vi "PH_Beckhoff_Watchdog.ProcCases.vi"(0 "i ref in":refnum<vi>, 1 "selector":string, 2 "Data":T1, 3 "call cluster":T2={"Object"="", "Selector"="", "CallType"=enum."synchronous", "Async Object"="", "Async Selector"="", "Data Descriptor"="", "Data"=[], "Error #"=0, "Expire"=0}, 5 "error in (no error)":errorcluster) -> (14 "i ref out":refnum<vi>, 17 "answer cluster":T2={"Object"="", "Selector"="", "CallType"=enum."synchronous", "Async Object"="", "Async Selector"="", "Data Descriptor"="", "Data"=[], "Error #"=0, "Expire"=0}, 19 "error out":errorcluster)   [LabVIEW 2014, in "PH_Beckhoff_Watchdog.lvlib"]
doc: "This method is called by a process from within the default case in the event loop. The methods of a class that are linked to events will be called from THIS method. Add your code here."
uses:
  PH_Beckhoff_Watchdog.lvlib
  CSCore/CSSystem/CoreDefs/CoreDefs.call_type.ctl
  CSCore/BaseProcess/BaseProcess.descriptor string definition.ctl
  CSCore/CSSystem/CoreDefs/CoreDefs.rawDataType.ctl
  CSCore/CSSystem/CoreLib/CoreLib.string 2 byte array.vi
  CSCore/BaseProcess/BaseProcess.lvlib
  CSCore/CSSystem/CoreLib/CoreLib.lvlib
  CSCore/CAEObj/CAEObj.lvlib
  PH_Common/PH_Common.lvlib
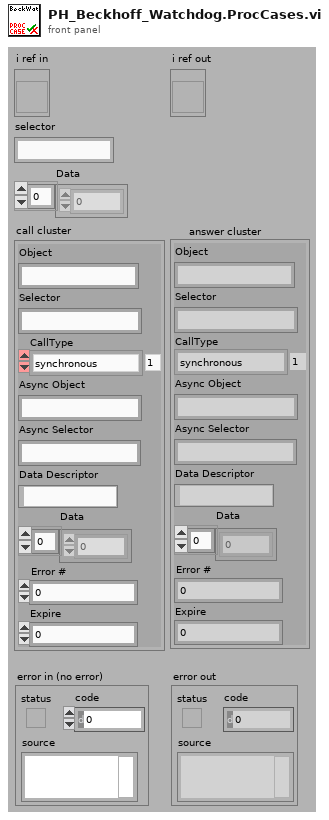
[diagram p1: front panel]
types:
  T1 = typedef "CoreDefs.rawDataType.ctl" = i8[]
  T2 = typedef "CoreDefs.call_type.ctl" = cluster{"Object":string, "Selector":string, "CallType":enum16{"simple", "synchronous", "asynchronous"}, "Async Object":string, "Async Selector":string, "Data Descriptor":T3, "Data":T1, "Error #":i32, "Expire":u32}
  T3 = typedef "BaseProcess.lvlib/BaseProcess.descriptor string definition.ctl" = string
  T4 = typedef "PH_StatusHandler.lvlib/PH_StatusHandler.Status.ctl" = i16
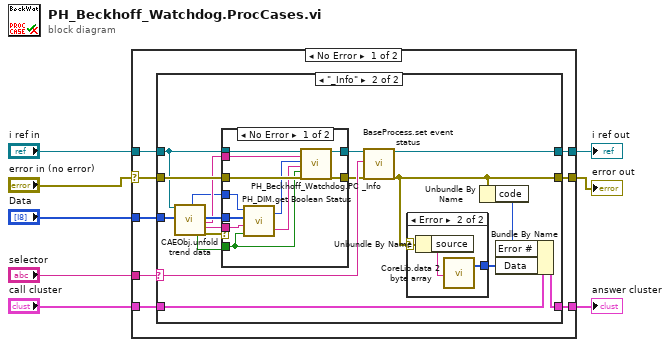
[diagram p0: block diagram]
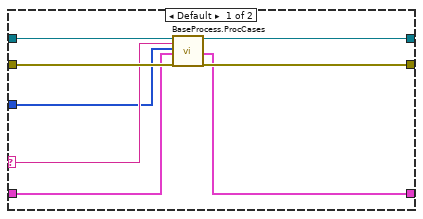
[diagram p2: hidden frame]
diagram:
  n1 = case shown="No Error" "error in (no error)" {
    selector: "error in (no error)" -> [w9 w60]
    tunnel: "selector" -> [w16 _]
    tunnel: [w15 w59] -> w7
    tunnel: "call cluster" -> [w14 w59]
    tunnel: "i ref in" -> [w13 w61]
    tunnel: [w12 w61] -> w4
    tunnel: [w11 w60] -> w3
    tunnel: "Data" -> [w10 _]
    frame No Error {
      n2 = case shown="\"_Info\"" w16 {
        selector: w16 -> [w19 w41]
        tunnel: w13 -> [w18 w31]
        tunnel: [w24 w40] -> w12
        tunnel: w14 -> [w20 w38]
        tunnel: [w21 w37] -> w15
        tunnel: w9 -> [w23 w36]
        tunnel: [w22 w39] -> w11
        tunnel: w10 -> [w17 w32]
        frame Default {
          n3 = call "BaseProcess.ProcCases.vi"("i ref in"=w18, "selector"=w19, "Data"=w17, "call cluster"=w20, "error in (no error)"=w23) -> ("i ref out"=w24:refnum<vi>, "answer cluster"=w21:T2, "error out"=w22:errorcluster)  [unwired: 12 in]
        }
        frame "_Info" {
          n4 = call "CAEObj.unfold trend data.vi"("i ref in"=w31, "raw trend data"=w32) -> ("quality"=w26:i32, "no link"=w28:bool, "data"=w29:i8[], "serviceName"=w27:string, "typeDescriptor"=w25:string, "error out"=w30:errorcluster)  [unwired: 9 in, 3 out]
          n5 = case shown="No Error" w30 {
            tunnel: w36 -> [w53 w54]
            tunnel: [w52 w55] -> w35
            tunnel: [w51 w54] -> w34
            tunnel: w31 -> [w50 w55]
            tunnel: w25 -> [w49 _]
            tunnel: w29 -> [w48 _]
            tunnel: w28 -> [w43 _]
            tunnel: w27 -> [w47 _]
            tunnel: w26 -> [w46 _]
            frame No Error {
              n6 = call "PH_DIM.get Boolean Status.vi"("no link"=w43, "typeDescriptor"=w49, "data"=w48, "quality"=w46) -> ("further information"=w45:string, "Status"=w44:T4)
              n7 = call "PH_Beckhoff_Watchdog.PC _Info.vi"("i ref in"=w50, "serviceName"=w47, "Status"=w44, "Further Information"=w45, "no link"=w43, "error in"=w53) -> ("i ref out"=w52:refnum<vi>, "error out"=w51:errorcluster)  [unwired: 12 in]
            }
            frame Error {
            }
          }
          n8 = call "BaseProcess.set event status.vi"("i ref in"=w35, "EventStatus"=w41, "error in (no error)"=w34) -> ("i ref out"=w40:refnum<vi>, "error out"=w39:errorcluster)  [unwired: 14 in, 1 out]
          n9 = case shown="Error" w39 {
            selector: w39 -> [_ w58]
            tunnel: [_ w56] -> w42
            frame No Error {
            }
            frame Error {
              n10 = Unbundle By Name(w58) -> ("source"=w57:string)
              n11 = call-poly "CoreLib.data 2 byte array.vi"("string"=w57) -> ("byteArray out"=w56:T1)  [unwired: 18 in]
            }
          }
          n12 = Unbundle By Name(w39) -> ("code"=w33:i32)
          n13 = Bundle By Name(cluster=w38, "Error #"=w33, "Data"=w42) -> (w37:T2)
        }
      }
    }
    frame Error {
    }
  }
  "answer cluster" <- w7
  "i ref out" <- w4
  "error out" <- w3
